vi "WS1021 ADI Read 64 DUT.vi"(6 "DUT Mask Mode (All)":T1=enum."All", 7 "FPGA":T2, 8 "Error In":errorcluster) -> (0 "Error Out":errorcluster, 3 "AD7747 Values":string[][](table))   [LabVIEW 2017]
uses:
  WS_VCAP Driver 039/Source/WSVCAP Shell/Type Defs/WSVCAP SHL FPGA Enum.ctl
  WS_VCAP Driver 039/Source/WSVCAP Shell/Type Defs/WSVCAP SHL I2C DUT Mask Mode Enum.ctl
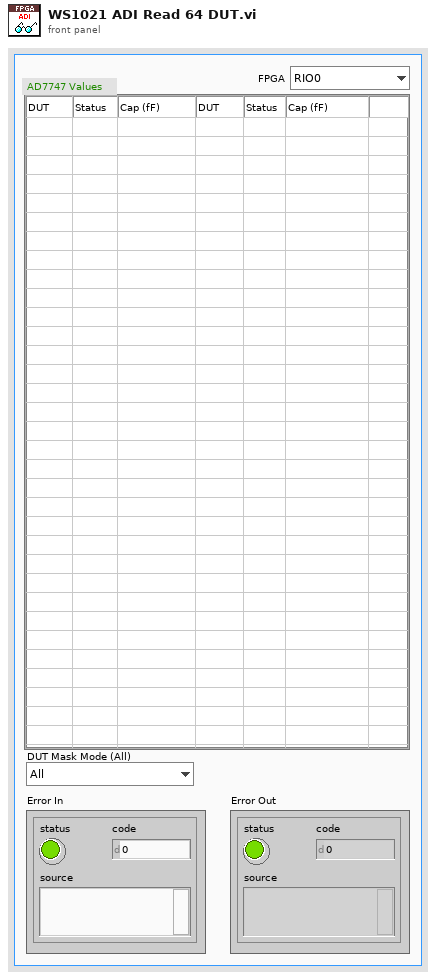
[diagram p1: front panel]
types:
  T1 = typedef "WSVCAP SHL I2C DUT Mask Mode Enum.ctl" = enum16{"Custom", "All"}
  T2 = typedef "WSVCAP SHL FPGA Enum.ctl" = enum16{"RIO0", "RIO1"}
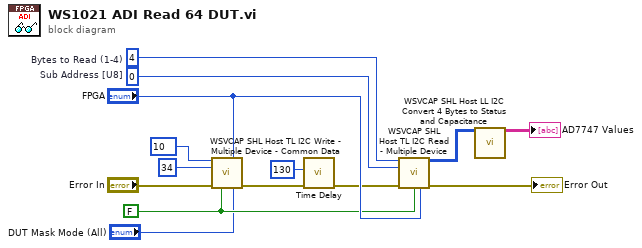
[diagram p0: block diagram]
diagram:
  w11 = u8 4  # Bytes to Read (1-4)
  w12 = u8 0  # Sub Address [U8]
  w4 = FALSE ("Log (T)")
  n1 = call "WSVCAP SHL Host TL I2C Write - Multiple Device - Common Data.vi"("Sub Address"=u8 10, "FPGA"="FPGA", "Data Out [U8]"=u8 34, "error in"="Error In", "Log (T)"=w4, "DUT Mask Mode (All)"="DUT Mask Mode (All)") -> ("error out"=w7:errorcluster)  [unwired: 9 in]
  n2 = call "Time Delay.vi"("Error In"=w7, "Delay(ms)"=u32 130) -> ("Error Out"=w5:errorcluster)  [unwired: 9 in]
  n3 = call "WSVCAP SHL Host TL I2C Read - Multiple Device.vi"("Bytes to Read (1-4)"=w11, "Sub Address [U8]"=w12, "error in"=w5, "Log (T)"=w4, "FPGA"="FPGA") -> ("C:1-64 Read Data [U8]"=w10:u8[][], "error out"=→"Error Out":errorcluster)  [unwired: 9 in]
  n4 = call "WSVCAP SHL Host LL I2C Convert 4 Bytes to Status and Capacitance.vi"("C:1-64 Read Data [U8]"=w10) -> ("AD7747 Values"=→"AD7747 Values":string[][])  [unwired: 14 in]
